vi "controlActorSensitivity.vi"(7 "Set":bool, 8 "error in":errorcluster, 9 "Sensitivity [0...7]":i32, 10 "axis in":u8, 11 "connection ID":refnum<k5>) -> (0 "error out":errorcluster, 1 "Sensitivity out":i32, 2 "axis out":i32, 3 "connection ID":refnum<k5>)   [LabVIEW 2016]
doc: "This VI retrieves or sets the sensitivity parameter of the currently connected positioner. The sensitivity affects the velocity, the positioner approaches a target position. The higher the sensitivity, the lower the velocity."
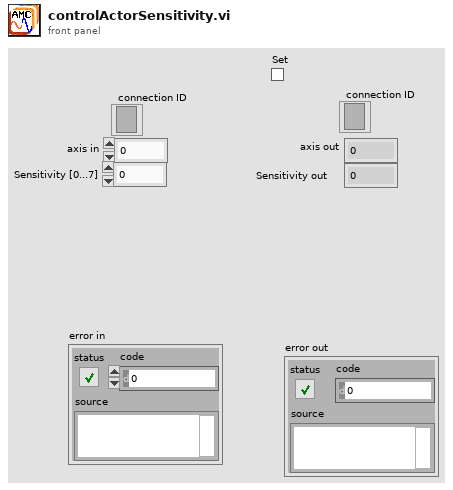
[diagram p1: front panel]
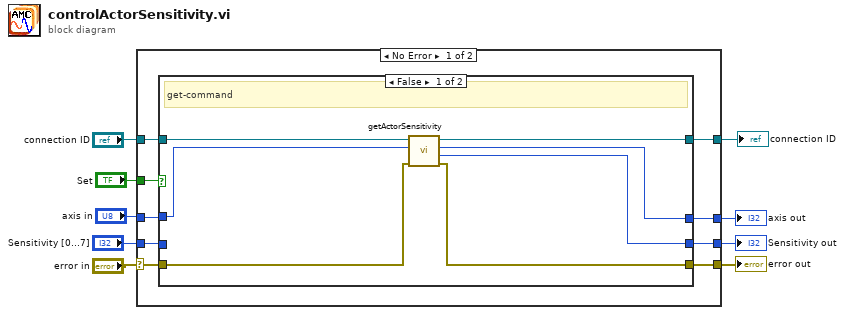
[diagram p0: block diagram]
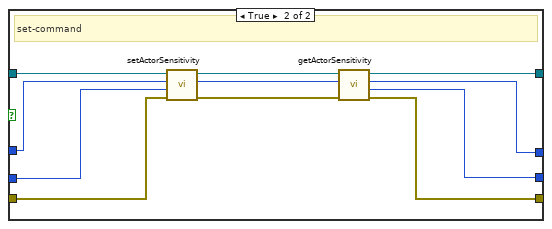
[diagram p2: hidden frame]
diagram:
  n1 = case shown="No Error" "error in" {
    selector: "error in" -> [w12 w40]
    tunnel: "axis in" -> [w18 w37]
    tunnel: [w16 w40] -> w8
    tunnel: "Sensitivity [0...7]" -> [w14 w38]
    tunnel: [w11 w38] -> w1
    tunnel: "Set" -> [w13 _]
    tunnel: [w15 w39] -> w6
    tunnel: "connection ID" -> [w17 w39]
    tunnel: [w10 w37] -> w2
    frame No Error {
      n2 = case shown="False" w13 {
        tunnel: [w20 w26] -> w15
        tunnel: w17 -> [w22 w36]
        tunnel: w18 -> [w23 w35]
        tunnel: [w24 w29] -> w16
        tunnel: w14 -> [_ w34]
        tunnel: w12 -> [w25 w33]
        tunnel: [w19 w28] -> w11
        tunnel: [w21 w27] -> w10
        frame False {
          # "get-command"
          n3 = call "getActorSensitivity.vi"("error in"=w25, "axis"=w23, "connection ID"=w22) -> ("error out"=w24:errorcluster, "sensitivity"=w19:i32, "axis_out"=w21:i32, "connection ID"=w20:refnum<k5>)  [unwired: 5 in]
        }
        frame True {
          # "set-command"
          n4 = call "setActorSensitivity.vi"("error in"=w33, "sensitivity"=w34, "axis"=w35, "connection ID"=w36) -> ("error out"=w30:errorcluster, "axis_out"=w31:i32, "connection ID"=w32:refnum<k5>)  [unwired: 5 in]
          n5 = call "getActorSensitivity.vi"("error in"=w30, "axis"=w31, "connection ID"=w32) -> ("error out"=w29:errorcluster, "sensitivity"=w28:i32, "axis_out"=w27:i32, "connection ID"=w26:refnum<k5>)  [unwired: 5 in]
        }
      }
    }
    frame Error {
    }
  }
  "error out" <- w8
  "axis out" <- w2
  "connection ID" <- w6
  "Sensitivity out" <- w1
